vi "SetSync.vi"(8 "error in":errorcluster, 10 "SyncMode":T1(ring), 11 "Port":refnum<visa-resource-name>) -> (0 "error out":errorcluster, 3 "Port out":refnum<visa-resource-name>)   [LabVIEW 2018]
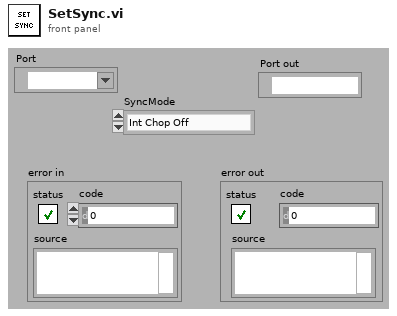
[diagram p1: front panel]
types:
  T1 = enum16{"Int Chop Off", "Int Chop On", "Ext Chop Off", "Ext Chop On"}
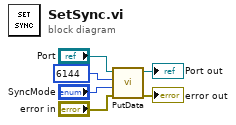
[diagram p0: block diagram]
diagram:
  n1 = call "PutData.vi"("error in"="error in", "Value"="SyncMode", "Location"=u32 6144, "Port"="Port") -> ("error out"=→"error out":errorcluster, "Port out"=→"Port out":refnum<visa-resource-name>)  [unwired: 6 in]
